vi "WPI_PWMOpen.vi"(8 "error in":errorcluster, 10 "PWM Channel":T2) -> (0 "error out":errorcluster, 3 "PWMDeviceRef":T1)   [LabVIEW 2017]
doc: "Opens a reference to the PWM port you specify. You must open a reference before using any other PWM VIs. After you open a reference to the PWM, you can use the Close VI to close the reference. The Open VI on the PWM palette opens references to custom motor controllers. You must use the Open VI on the RobotDrive or MotorControl palettes to open references to those devices. For example, use the Jaguar instance of the Open VI on the MotorControl palette to open a reference to the Jaguar motor controller.\n\nThis software is licensed. Open the labview\\readme\\WPI Robotics Library Open Source License.txt file for more information."
uses:
  <vilib>/Rock Robotics/SystemInterfaces/DIO/FPGA_DIOPWMChannel.ctl
  <vilib>/Rock Robotics/WPI/PWM/WPI_PWMDeviceRef.ctl
  <vilib>/Rock Robotics/WPI/PWM/WPI_PWMChannelCacheOp.ctl
  <vilib>/Rock Robotics/SystemInterfaces/NetworkCommunication/NetComm_UsageReport_ResourceType.ctl
  <vilib>/Rock Robotics/SystemInterfaces/System/FPGA_SystemGet.vi
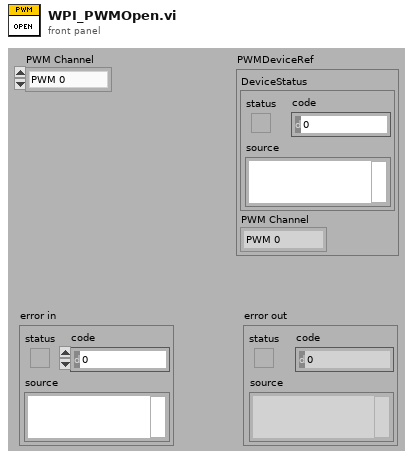
[diagram p1: front panel]
types:
  T1 = typedef "WPI_PWMDeviceRef.ctl" = cluster{"DeviceStatus":errorcluster, "PWM Channel":T2}
  T2 = typedef "FPGA_DIOPWMChannel.ctl" = enum8{"PWM 0", "PWM 1", "PWM 2", "PWM 3", "PWM 4", "PWM 5", "PWM 6", "PWM 7", "PWM 8", "PWM 9", "PWM MXP 0", "PWM MXP 1", "PWM MXP 2", "PWM MXP 3", "PWM MXP 4", "PWM MXP 5", "PWM MXP 6", "PWM MXP 7", "PWM MXP 8", "PWM MXP 9", "Invalid"}
  T3 = typedef "NetComm_UsageReport_ResourceType.ctl" = enum8{"Controller", "Module", "Language", "CANPlugin", "Accelerometer", "ADXL345", "AnalogChannel", "AnalogTrigger", "AnalogTriggerOutput", "CANJaguar", "Compressor", "Counter", "Dashboard", "DigitalInput", "DigitalOutput", "DriverStationCIO", "DriverStationEIO", "DriverStationLCD", "Encoder", "GearTooth", "Gyro", "I2C", "Framework", "Jaguar", "Joystick", "Kinect", "KinectStick", "PIDController", "Preferences", "PWM", "Relay", "RobotDrive", "SerialPort", "Servo", "Solenoid", "SPI", "Task", "Ultrasonic", "Victor", "Button", "Command", "AxisCamera", "PCVideoServer", "SmartDashboard", "Talon", "HiTechnicColorSensor", "HiTechnicAccel", "HiTechnicCompass", "SRF08", "AnalogOutput", "Victor SP", "Talon SRX", "CAN Talon SRX", "ADXL362 Accel", "ADXRS450 Gyro", "Rev SPARK", "Mindsensors SD540", "Digital Filter", "ADIS16448", "PDP", "PCM", "PigeonIMU", "Nidec Brushless", "CTRE CANifier", "CTRE Future 0", "CTRE Future 1", "CTRE Future 2", "CTRE Future 3", "CTRE Future 4", "CTRE Future 5", "CTRE Future 6"}
  T4 = typedef "WPI_PWMChannelCacheOp.ctl" = enum16{"Acquire", "Release", "Status"}
  T5 = typedef "WPI_DigitalModuleDeviceRef.ctl" = cluster{"DevStatus":errorcluster}
  T6 = typedef "FPGA_DIODevRef.ctl" = cluster{"DevStatus":errorcluster}
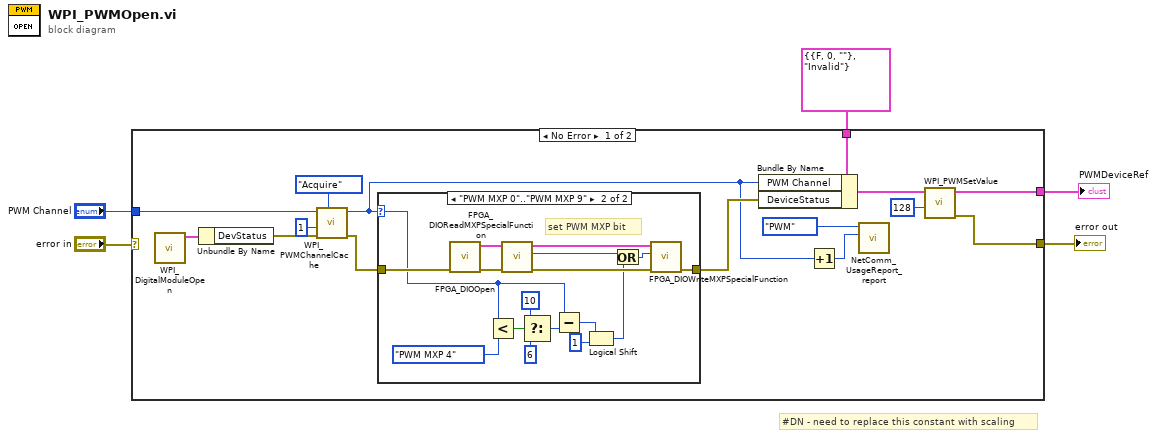
[diagram p0: block diagram]
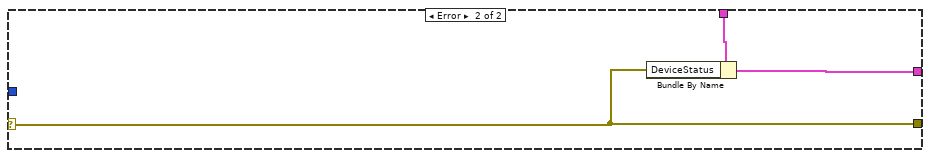
[diagram p3: hidden frame]
diagram:
  # "#DN - need to replace this constant with scaling"
  n1 = case shown="No Error" "error in" {
    selector: "error in" -> [_ w39]
    tunnel: "PWM Channel" -> [w18 _]
    tunnel: T1 {"DeviceStatus"={"status"=FALSE, "code"=0, "source"=""}, "PWM Channel"=enum."Invalid"} ("PWMDeviceRef") -> [w19 w41]
    tunnel: [w14 w40] -> w2
    tunnel: [w13 w39] -> w3
    frame No Error {
      n2 = call <vilib>:"WPI_DigitalModuleOpen.vi"() -> ("DigitalModuleDevRef"=w17:T5)  [unwired: 2 in, 9 out]
      n3 = Unbundle By Name(w17) -> ("DevStatus"=w16:errorcluster)
      n4 = call <vilib>:"WPI_PWMChannelCache.vi"("Operation"=WPI_PWMChannelCacheOp."Acquire", "error in (no error)"=w16, "Additional Depth"=1, "PWMChannel"=w18) -> ("error out"=w9:errorcluster, "AllocatedPWMChannel"=w7:T2)  [unwired: 1 in, 5 out]
      n5 = case shown="\"PWM MXP 0\"..\"PWM MXP 9\"" w7 {
        selector: w7 -> [_ w23]
        tunnel: w9 -> [w21 w33]
        tunnel: [w21 w32] -> w8
        frame Default {
        }
        frame "PWM MXP 0".."PWM MXP 9" {
          # "set PWM MXP bit"
          n6 = call <vilib>:"FPGA_DIOOpen.vi"("error in (no error)"=w33) -> ("error out"=w37:errorcluster, "DIODeviceRef"=w38:T6)  [unwired: 9 out]
          n7 = Less?(x=w23, y=FPGA_DIOPWMChannel."PWM MXP 4" ("PWM Channel")) -> (x < y?=w25:bool)
          n8 = call <vilib>:"FPGA_DIOReadMXPSpecialFunction.vi"("error in (no error)"=w37, "DIODeviceRef In"=w38) -> ("error out"=w31:errorcluster, "EnableSpecialFunction"=w35:u16, "DIODeviceRef Out"=w36:T6)  [unwired: 7 in]
          n9 = Select(t=u16 10 ("EnableSpecialFunction"), s=w25, f=u16 6 ("EnableSpecialFunction")) -> (s? t:f=w27:u16)
          n10 = Subtract(x=w23, y=w27) -> (x-y=w30:u16)
          n11 = Logical Shift(y=w30, x=u16 1) -> (x << y=w22:u16)
          n12 = Or(x=w35, y=w22) -> (x .or. y?=w34:u16)
          n13 = call <vilib>:"FPGA_DIOWriteMXPSpecialFunction.vi"("error in (no error)"=w31, "EnableSpecialFunction"=w34, "DIODeviceRef In"=w36) -> ("error out"=w32:errorcluster)  [unwired: 7 in, 1 out]
        }
      }
      n14 = Bundle By Name(cluster=w19, "PWM Channel"=w7, "DeviceStatus"=w8) -> (w15:T1)
      n15 = Increment(x=w7) -> (x+1=w10:T2)
      n16 = call <vilib>:"NetComm_UsageReport_report.vi"("Instance Number"=w10, "Resource Type"=NetComm_UsageReport_ResourceType."PWM") -> ()  [unwired: 10 in]
      n17 = call <vilib>:"WPI_PWMSetValue.vi"("Value"=u8 128, "PWMDeviceRef"=w15) -> ("error out"=w13:errorcluster, "PWMDeviceRef"=w14:T1)  [unwired: 2 in, 6 out]
    }
    frame Error {
      n18 = Bundle By Name(cluster=w41, "DeviceStatus"=w39) -> (w40:T1)
    }
  }
  "PWMDeviceRef" <- w2
  "error out" <- w3
